vi "配置初始化.vi"(8 "error in (no error)":errorcluster) -> (0 "error out":errorcluster)   [LabVIEW 2016]
uses:
  <vilib>/Utility/config.llb/NI_LVConfig.lvlib
  API/OpSignIn/opSignIn.lvlib
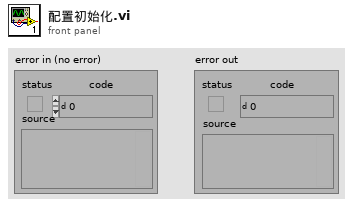
[diagram p1: front panel]
types:
  T1 = typedef "NI_LVConfig.lvlib/Config Data RefNum.ctl" = refnum<k1>
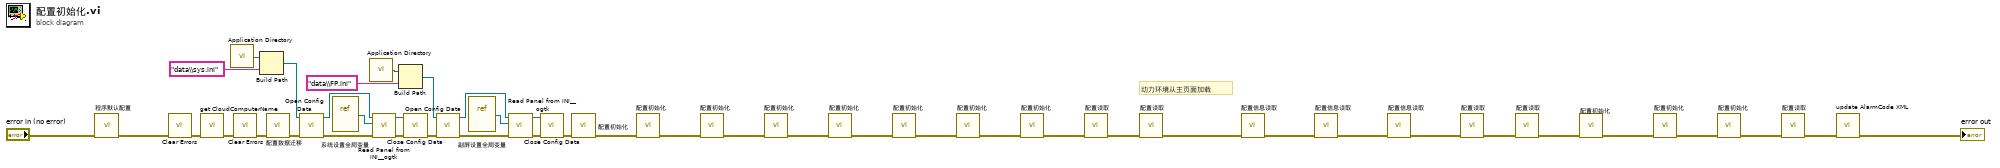
[diagram p0: block diagram]
diagram:
  # "动力环境从主页面加载"
  n1 = call "程序默认配置.vi"("error in (no error)"="error in (no error)") -> ("error out"=w4:errorcluster)  [unwired: 10 in]
  n2 = call <vilib>:"Clear Errors.vi"("error in (no error)"=w4) -> ("error out"=w3:errorcluster)  [unwired: 5 in, 1 out]
  n3 = call "get CloudComputerName.vi"("error in (no error)"=w3) -> ("error out"=w17:errorcluster)  [unwired: 9 in, 1 out]
  n4 = call <vilib>:"Application Directory.vi"() -> ("Application Directory"=w35:path)
  n5 = call <vilib>:"Clear Errors.vi"("error in (no error)"=w17) -> ("error out"=w9:errorcluster)  [unwired: 5 in, 1 out]
  n6 = Build Path(base path=w35, name or relative path="data\\sys.ini" ("名称或相对路径")) -> (appended path=w37:path)
  n7 = call "配置数据迁移.vi"("error in (no error)"=w9) -> ("error out"=w29:errorcluster)  [unwired: 10 in]
  n8 = call <vilib>:"Open Config Data.vi"("error in (no error)"=w29, "configuration file path"=w37) -> ("error out"=w30:errorcluster, "refnum"=w31:T1)  [unwired: 7 in, 1 out]
  n9 = vi-ref "系统设置全局变量.vi"() -> (w32:refnum<vi>)
  n10 = call <vilib>:"Application Directory.vi"() -> ("Application Directory"=w21:path)
  n11 = call <userlib>:"Read Panel from INI__ogtk.vi"("error in (no error)"=w30, "VI ref"=w32, "refnum"=w31) -> ("error out"=w33:errorcluster, "refnum out"=w34:T1)  [unwired: 7 in]
  n12 = Build Path(base path=w21, name or relative path="data\\FP.ini" ("名称或相对路径")) -> (appended path=w27:path)
  n13 = call <vilib>:"Close Config Data.vi"("error in (no error)"=w33, "refnum"=w34) -> ("error out"=w20:errorcluster)  [unwired: 8 in, 1 out]
  n14 = call <vilib>:"Open Config Data.vi"("error in (no error)"=w20, "configuration file path"=w27) -> ("error out"=w26:errorcluster, "refnum"=w23:T1)  [unwired: 7 in, 1 out]
  n15 = vi-ref "副屏设置全局变量.vi"() -> (w24:refnum<vi>)
  n16 = call <userlib>:"Read Panel from INI__ogtk.vi"("error in (no error)"=w26, "VI ref"=w24, "refnum"=w23) -> ("error out"=w25:errorcluster, "refnum out"=w22:T1)  [unwired: 7 in]
  n17 = call <vilib>:"Close Config Data.vi"("error in (no error)"=w25, "refnum"=w22) -> ("error out"=w19:errorcluster)  [unwired: 8 in, 1 out]
  n18 = call "配置初始化.vi"("error in (no error)"=w19) -> ("error out"=w44:errorcluster)  [unwired: 10 in]
  n19 = call "配置初始化.vi"("error in (no error)"=w44) -> ("error out"=w43:errorcluster)  [unwired: 10 in]
  n20 = call "配置初始化.vi"("error in (no error)"=w43) -> ("error out"=w42:errorcluster)  [unwired: 10 in]
  n21 = call "配置初始化.vi"("error in (no error)"=w42) -> ("error out"=w41:errorcluster)  [unwired: 10 in]
  n22 = call "配置初始化.vi"("error in (no error)"=w41) -> ("error out"=w40:errorcluster)  [unwired: 10 in]
  n23 = call "配置初始化.vi"("error in (no error)"=w40) -> ("error out"=w39:errorcluster)  [unwired: 10 in]
  n24 = call "配置初始化.vi"("error in (no error)"=w39) -> ("error out"=w38:errorcluster)  [unwired: 10 in]
  n25 = call "配置初始化.vi"("error in (no error)"=w38) -> ("error out"=w10:errorcluster)  [unwired: 10 in]
  n26 = call "配置读取.vi"("error in (no error)"=w10) -> ("error out"=w16:errorcluster)  [unwired: 10 in]
  n27 = call "配置读取.vi"("error in (no error)"=w16) -> ("error out"=w15:errorcluster)  [unwired: 10 in]
  n28 = call "配置信息读取.vi"("error in (no error)"=w15) -> ("error out"=w14:errorcluster)  [unwired: 10 in]
  n29 = call "配置信息读取.vi"("error in (no error)"=w14) -> ("error out"=w13:errorcluster)  [unwired: 10 in]
  n30 = call "配置信息读取.vi"("error in (no error)"=w13) -> ("error out"=w12:errorcluster)  [unwired: 10 in]
  n31 = call "配置读取.vi"("error in (no error)"=w12) -> ("error out"=w11:errorcluster)  [unwired: 10 in]
  n32 = call "配置读取.vi"("error in (no error)"=w11) -> ("error out"=w2:errorcluster)  [unwired: 10 in]
  n33 = call "配置初始化.vi"("error in (no error)"=w2) -> ("error out"=w1:errorcluster)  [unwired: 10 in]
  n34 = call "配置初始化.vi"("error in (no error)"=w1) -> ("错误输出"=w8:errorcluster)  [unwired: 10 in]
  n35 = call "配置初始化.vi"("error in (no error)"=w8) -> ("error out"=w5:errorcluster)  [unwired: 10 in]
  n36 = call "配置读取.vi"("error in (no error)"=w5) -> ("error out"=w6:errorcluster)  [unwired: 10 in]
  n37 = call "update AlarmCode XML.vi"("error in (no error)"=w6) -> ("error out"=→"error out":errorcluster)  [unwired: 10 in]
